vi "GE5565 DMA Polling Write and Read (DBL) Example (Cluster) mod.vi"() -> ()   [LabVIEW 2011]
uses:
  <instrlib>/GE 5565 PIORC/Public/GE5565 Write (U32) Cluster.vi
  <instrlib>/GE 5565 PIORC/Public/DMA/GE5565 DMA Read (U64) Cluster.vi
  <instrlib>/GE 5565 PIORC/GE 5565 PIORC.lvlib
panel:
  in  "offset (0)":u32
  out "error out":errorcluster
  in  "VISA resource name (empty)":refnum<visa-resource-name>
  out "Data from RM":dbl[](array[numeric])
  in  "Data to Write":dbl[](array[numeric])=[1.0, 2.0, 3.0, 4.0, 5.0]
  in  "transfer size (1024 bytes)":u32=5
  in  "stop":bool
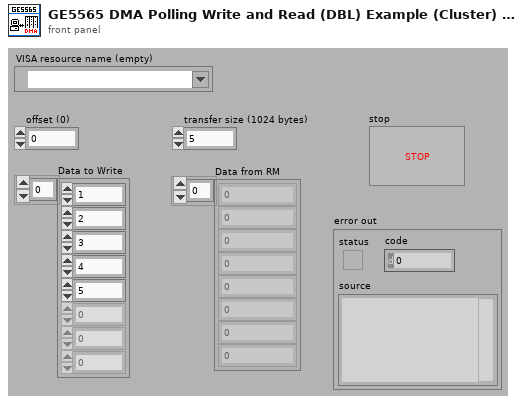
[diagram p1: front panel]
types:
  T1 = cluster{"VMIC 5565 Resource":refnum<visa-resource-name>, "MEMACC Resource":refnum<visa-resource-name>, "byte count":u32, "mem offset":u32}
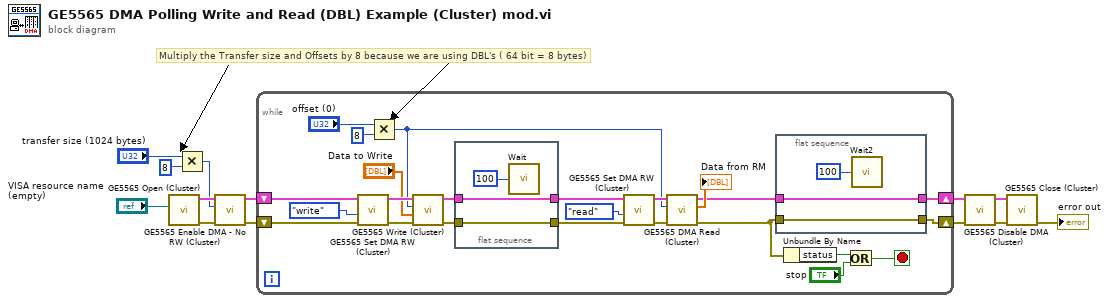
[diagram p0: block diagram]
diagram:
  # "Multiply the Transfer size and Offsets by 8 because we are using DBL's ( 64 bit = 8 bytes)"
  n1 = call <instrlib>:"GE5565 Open (Cluster).vi"("VISA resource name (empty)"="VISA resource name (empty)") -> ("error out"=w12:errorcluster, "VMIC-5565"=w13:T1)  [unwired: 2 in, 3 out]
  n2 = Multiply(x="transfer size (1024 bytes)", y=u32 8) -> (x*y=w2:u32)
  n3 = call <instrlib>:"GE5565 Enable DMA - No RW (Cluster).vi"("error in (no error)"=w12, "transfer size (1024 bytes)"=w2, "VMIC-5565"=w13) -> ("error out"=w10:errorcluster, "VMIC-5565"=w11:T1)  [unwired: 3 out]
  n4 = while {
    shift-right: [w19] -> w8
    shift-left: w10 -> [w34]
    shift-right: [w21] -> w9
    shift-left: w11 -> [w35]
    stop <- w36 stop-if-true
    n5 = call <instrlib>:"GE5565 Set DMA RW (Cluster).vi"("error in (no error)"=w34, "operation (read)"=enum16{"read", "write"}."write", "VMIC-5565"=w35) -> ("error out"=w31:errorcluster, "VMIC-5565"=w32:T1)  [unwired: 3 out]
    n6 = Multiply(x="offset (0)", y=u32 8) -> (x*y=w16:u32)
    n7 = call-poly <instrlib>:"GE5565 Write (Cluster).vi"("error in (no error)"=w31, "buffer"="Data to Write", "offset (0)"=w16, "VMIC reference in"=w32) -> ("error out"=w28:errorcluster, "VMIC reference out"=w29:T1)  [unwired: 2 out]
    n8 = flat-sequence {
      tunnel: w29 -> [w42]
      tunnel: w28 -> [w41]
      tunnel: [w42] -> w27
      tunnel: [w41] -> w26
      frame #0 {
        n9 = call "Wait"("Count(uSec)"=u32 100) -> ()  [unwired: 1 out]
      }
    }
    n10 = call <instrlib>:"GE5565 Set DMA RW (Cluster).vi"("error in (no error)"=w26, "operation (read)"=enum16{"read", "write"}."read", "VMIC-5565"=w27) -> ("error out"=w23:errorcluster, "VMIC-5565"=w24:T1)  [unwired: 3 out]
    n11 = call-poly <instrlib>:"GE5565 DMA Read (Cluster).vi"("error in (no error)"=w23, "offset (0)"=w16, "VMIC reference in"=w24) -> ("error out"=w14:errorcluster, "buffer"=→"Data from RM":dbl[], "VMIC reference out"=w20:T1)  [unwired: 2 out]
    n12 = flat-sequence {
      tunnel: [w40] -> w21
      tunnel: w20 -> [w40]
      tunnel: w14 -> [w39]
      tunnel: [w39] -> w19
      frame #0 {
        n13 = call "Wait2"("Count(uSec)"=u32 100) -> ()  [unwired: 1 out]
      }
    }
    n14 = Unbundle By Name(w14) -> ("status"=w15:bool)
    n15 = Or(x=w15, y="stop") -> (x .or. y?=w36:bool)
  }
  n16 = call <instrlib>:"GE5565 Disable DMA (Cluster).vi"("error in (no error)"=w8, "VMIC reference in"=w9) -> ("error out"=w6:errorcluster, "VMIC reference out"=w7:T1)  [unwired: 4 out]
  n17 = call <instrlib>:"GE5565 Close (Cluster).vi"("error in (no error)"=w6, "VMIC reference in"=w7) -> ("error out"=→"error out":errorcluster)  [unwired: 5 out]
